vi "move Z Relative.vi"(10 "Z Speed":u32, 11 "z mm":dbl) -> ()   [LabVIEW 2017]
uses:
  Settings/Traverse-Settings-Global.vi
  ICNC/ICNC2.lvlib
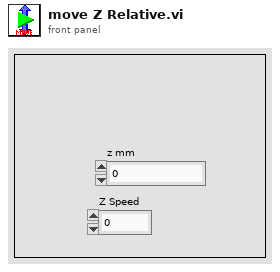
[diagram p1: front panel]
types:
  T1 = typedef "Settings-Control.ctl" = cluster{"Acceleration":dbl[], "Deceleration":dbl[], "Max Velocity":dbl[], "Speed":dbl, "Pulse/Degree":dbl, "Degre Factor":dbl[], "mm/rotation":dbl[], "Traverse Name":string}
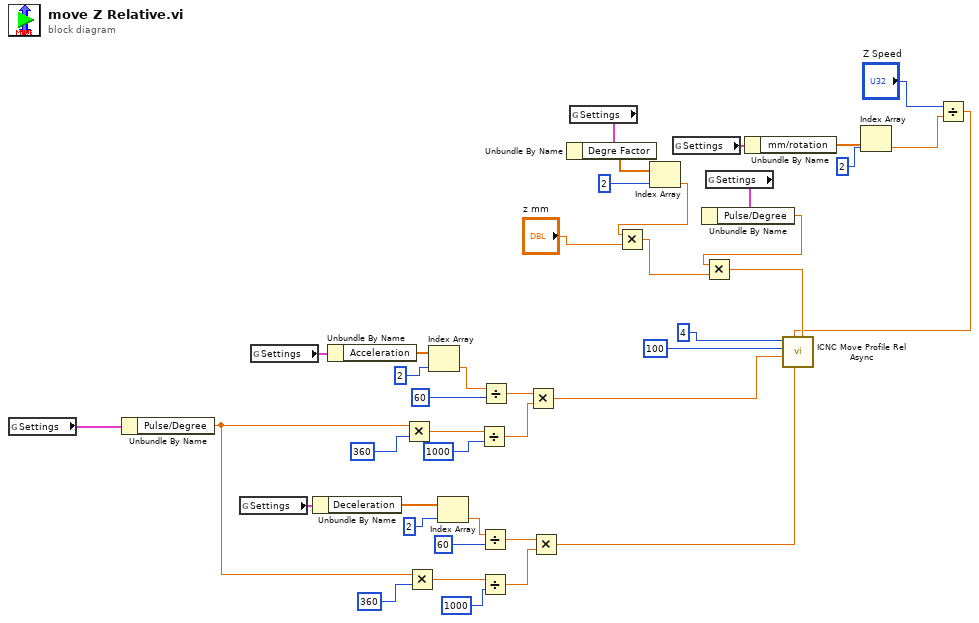
[diagram p0: block diagram]
diagram:
  n1 = global read "Traverse-Settings-Global.vi" "Settings"() -> (w23:T1)
  n2 = Unbundle By Name(w23) -> ("Pulse/Degree"=w22:dbl)
  n3 = global read "Traverse-Settings-Global.vi" "Settings"() -> (w17:T1)
  n4 = global read "Traverse-Settings-Global.vi" "Settings"() -> (w21:T1)
  n5 = Unbundle By Name(w17) -> ("Deceleration"=w16:dbl[])
  n6 = Unbundle By Name(w21) -> ("Acceleration"=w20:dbl[])
  n7 = Multiply(x=w22, y=360) -> (x*y=w31:dbl)
  n8 = Multiply(x=w22, y=360) -> (x*y=w30:dbl)
  n9 = Index Array(array=w20, index=2) -> (element=w18:dbl)
  n10 = Index Array(array=w16, index=2) -> (element=w14:dbl)
  n11 = Divide(x=w31, y=1000) -> (x/y=w41:dbl)
  n12 = Divide(x=w14, y=60) -> (x/y=w37:dbl)
  n13 = Divide(x=w30, y=1000) -> (x/y=w36:dbl)
  n14 = Divide(x=w18, y=60) -> (x/y=w32:dbl)
  n15 = Multiply(x=w32, y=w41) -> (x*y=w27:dbl)
  n16 = Multiply(x=w37, y=w36) -> (x*y=w26:dbl)
  n17 = global read "Traverse-Settings-Global.vi" "Settings"() -> (w12:T1)
  n18 = Unbundle By Name(w12) -> ("Degre Factor"=w10:dbl[])
  n19 = Index Array(array=w10, index=2) -> (element=w9:dbl)
  n20 = Multiply(x=w9, y="z mm") -> (x*y=w25:dbl)
  n21 = global read "Traverse-Settings-Global.vi" "Settings"() -> (w6:T1)
  n22 = global read "Traverse-Settings-Global.vi" "Settings"() -> (w13:T1)
  n23 = Unbundle By Name(w13) -> ("Pulse/Degree"=w8:dbl)
  n24 = Multiply(x=w8, y=w25) -> (x*y=w24:dbl)
  n25 = Unbundle By Name(w6) -> ("mm/rotation"=w5:dbl[])
  n26 = Index Array(array=w5, index=2) -> (element=w3:dbl)
  n27 = Divide(x="Z Speed", y=w3) -> (x/y=w1:dbl)
  n28 = call <menus>:"ICNC Move Profile Rel Async.vi"("Distance"=w24, "Decel"=w26, "Speed"=w1, "Accel"=w27, "FStartStop"=100, "Axe"=4) -> ()  [unwired: 4 in, 2 out]
